vi "Set Dichroic Position.vi"(0 "Notifier Name":string, 7 "Dichroic Position":i32, 11 "Error In":errorcluster) -> (4 "Notifier Name Dup":string, 8 "Position":i32, 13 "Error":bool, 15 "Error Out":errorcluster)   [LabVIEW 2020]
uses:
  Spinning Disk Type Defs/SD Notifer Data.ctl
  Spinning Disk Type Defs/SD Actions.ctl
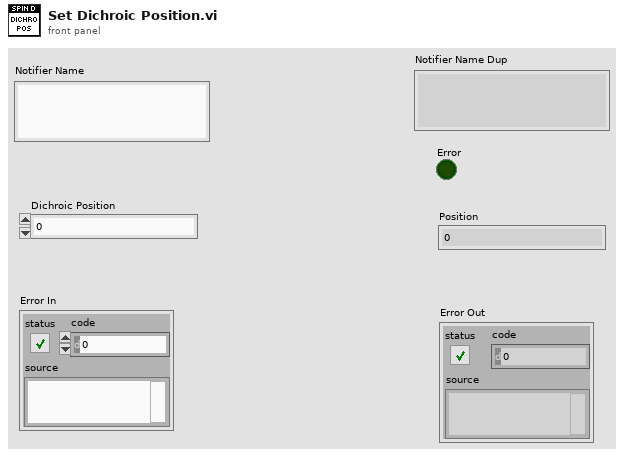
[diagram p1: front panel]
types:
  T1 = typedef "SD Notifer Data.ctl" = cluster{"Actions":T2, "Disk On?":bool, "Dichroic Pos.":i32, "Filter Wheel Pos.":i32, "Disk Pos.":i32, "Recived":bool, "Num Pos":i32[]}
  T2 = typedef "SD Actions.ctl" = enum16{"Status", "Get All Pos.", "Get Num. Pos.", "Home All", "Set Filter Wheel Pos.", "Set Disk Pos.", "Set Dichroic Pos.", "Disk On", "Disk Off", "Quit"}
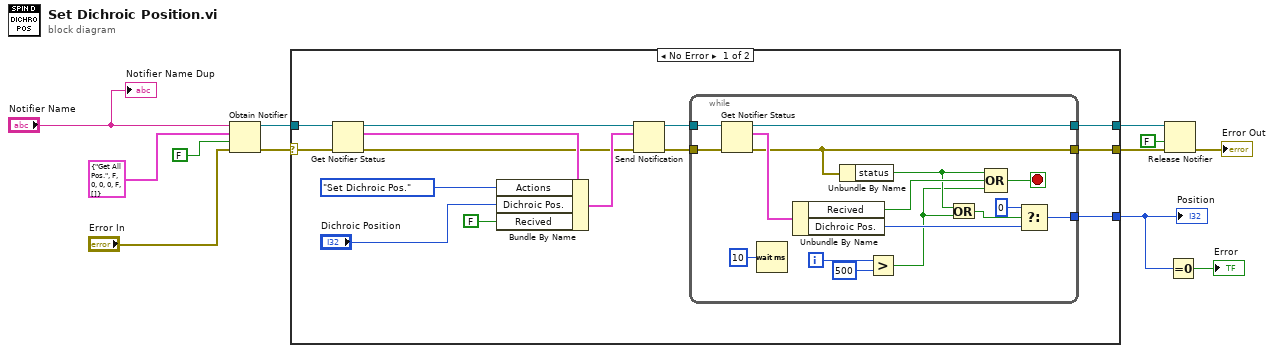
[diagram p0: block diagram]
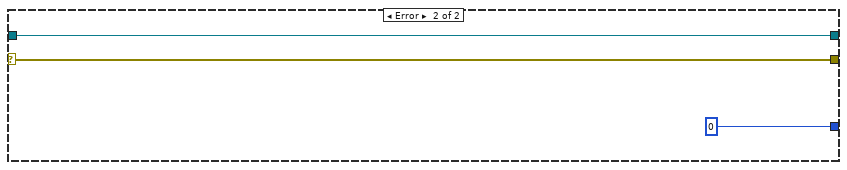
[diagram p2: hidden frame]
diagram:
  n1 = Obtain Notifier(name (unnamed)="Notifier Name", notification data type=T1 {"Actions"=enum."Get All Pos.", "Disk On?"=FALSE, "Dichroic Pos."=0, "Filter Wheel Pos."=0, "Disk Pos."=0, "Recived"=FALSE, "Num Pos"=[]} ("XLight Notifier Data"), create if not found? (T)=FALSE, error in (no error)="Error In") -> (notifier out=w8:refnum<notifier>, error out=w5:errorcluster)  [unwired: 1 out]
  n2 = case shown="No Error" w5 {
    selector: w5 -> [w25 w44]
    tunnel: w8 -> [w26 w45]
    tunnel: [w14 w45] -> w7
    tunnel: [w15 w44] -> w4
    tunnel: [w13 0 ("Filter Wheel Pos.")] -> w2
    frame No Error {
      n3 = Get Notifier Status(notifier=w26, error in (no error)=w25) -> (notifier out=w20:refnum<notifier>, current notification=w24:T1, error out=w18:errorcluster)  [unwired: 2 out]
      n4 = Bundle By Name(cluster=w24, "Actions"=SD_Actions."Set Dichroic Pos.", "Dichroic Pos."="Dichroic Position", "Recived"=FALSE) -> (w19:T1)
      n5 = Send Notification(notification=w19, notifier=w20, error in (no error)=w18) -> (notifier out=w17:refnum<notifier>, error out=w16:errorcluster)
      n6 = while {
        tunnel: w17 -> [w40]
        tunnel: w16 -> [w39]
        tunnel: [w30] -> w15
        tunnel: [w29] -> w14
        tunnel: [w28] -> w13
        i -> [w42]
        stop <- w31 stop-if-true
        n7 = Get Notifier Status(notifier=w40, error in (no error)=w39) -> (notifier out=w29:refnum<notifier>, current notification=w38:T1, error out=w30:errorcluster)  [unwired: 2 out]
        n8 = Wait (ms)(milliseconds to wait=u32 10) -> ()  [unwired: 1 out]
        n9 = Unbundle By Name(w38) -> ("Recived"=w37:bool, "Dichroic Pos."=w36:i32)
        n10 = Unbundle By Name(w30) -> ("status"=w34:bool)
        n11 = Greater?(x=w42, y=500) -> (0:w33:bool)
        n12 = Or(x=w34, y=w33) -> (x .or. y?=w32:bool)
        n13 = Compound Arithmetic op=OR(w34, w37, w33) -> (w31:bool)
        n14 = Select(t=0, s=w32, f=w36) -> (s? t:f=w28:i32)
      }
    }
    frame Error {
    }
  }
  "Position" <- w2
  n15 = Release Notifier(notifier=w7, force destroy? (F)=FALSE, error in (no error)=w4) -> (error out=→"Error Out":errorcluster)  [unwired: 2 out]
  n16 = Equal To 0?(x=w2) -> (x = 0?=→"Error":bool)
  "Notifier Name Dup" <- "Notifier Name"
